vi "PicoHandsOnExample.vi"() -> ()   [LabVIEW 2020]
doc: "Example that shows how to communicate with the Hands On Raspberry Pico board used during the CTI LabVIEW Training"
uses:
  <instrlib>/HandsOnPi2040/Public/DigIns.ctl
  <instrlib>/HandsOnPi2040/Public/AnaIns.ctl
  <instrlib>/HandsOnPi2040/Public/DigOuts.ctl
  <instrlib>/HandsOnPi2040/cti-drivers-lv-visa-main/CTI-Visa/Identity.ctl
  <instrlib>/HandsOnPi2040/Public/AOs.ctl
  <instrlib>/HandsOnPi2040/Public/PWMSettings.ctl
  <instrlib>/HandsOnPi2040/HandsOnPi2040.lvlib
  <instrlib>/HandsOnPi2040/cti-drivers-lv-visa-main/CTI-Visa/CTI-Visa.lvlib
panel:
  in  "Frequency":sgl(slide) scale=10.0..500000.0
  in  "Duty":sgl(slide) scale=0.0..1.0
  out "Identity":T1
  out "LoopIndex":i32
  in  "Digital Output":T2=enum."DO1 (GPIO2)"
  in  "DOBEEP":bool
  in  "DO4":bool
  in  "DO3":bool
  in  "DO2":bool
  out "AnInValue":u16(graph)
  in  "Analog Inputs":T3=enum."AI1 (GPIO26)"
  out "DIStatus":bool
  in  "Digital Inputs":T4=enum."DI1 (GPIO7)"
  out "DOStatus":bool
  in  "DO1":bool
  in  "VISA resource name":refnum<visa-resource-name>="TCPIP0::192.168.10.207::6430::SOCKET"
  out "error out":errorcluster
  in  "stop":bool
  # "READ"
  # "WRITE"
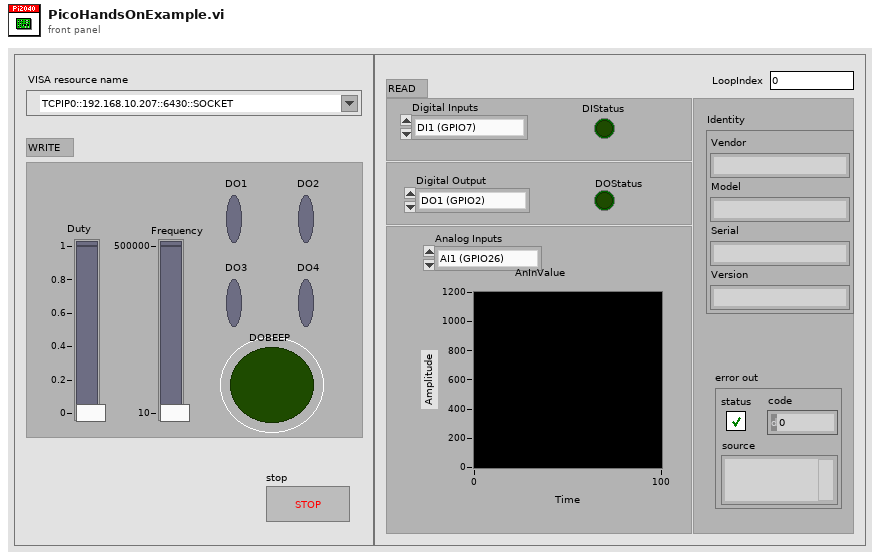
[diagram p1: front panel]
types:
  T1 = typedef "CTI-Visa.lvlib/Identity.ctl" = cluster{"Vendor":string, "Model":string, "Serial":string, "Version":string}
  T2 = typedef "HandsOnPi2040.lvlib/DigOuts.ctl" = enum16{"No DO - Error", "DO1 (GPIO2)", "DO2 (GPIO3)", "DO3 (GPIO4)", "DO4 (GPIO5)", "BEEP (GPIO6)"}
  T3 = typedef "HandsOnPi2040.lvlib/AnaIns.ctl" = enum16{"No AI - Error", "AI1 (GPIO26)", "AI2 (GPIO27)"}
  T4 = typedef "HandsOnPi2040.lvlib/DigIns.ctl" = enum16{"No DI - Error", "DI1 (GPIO7)", "DI2 (GPIO8)", "DI3 (GPIO9)", "DI4 (GPIO10)"}
  T5 = typedef "HandsOnPi2040.lvlib/PWMSettings.ctl" = cluster{"Duty":sgl, "Frequency":sgl}
  T6 = typedef "HandsOnPi2040.lvlib/AOs.ctl" = enum16{"No AO - Error", "AO1 (GPIO28)"}
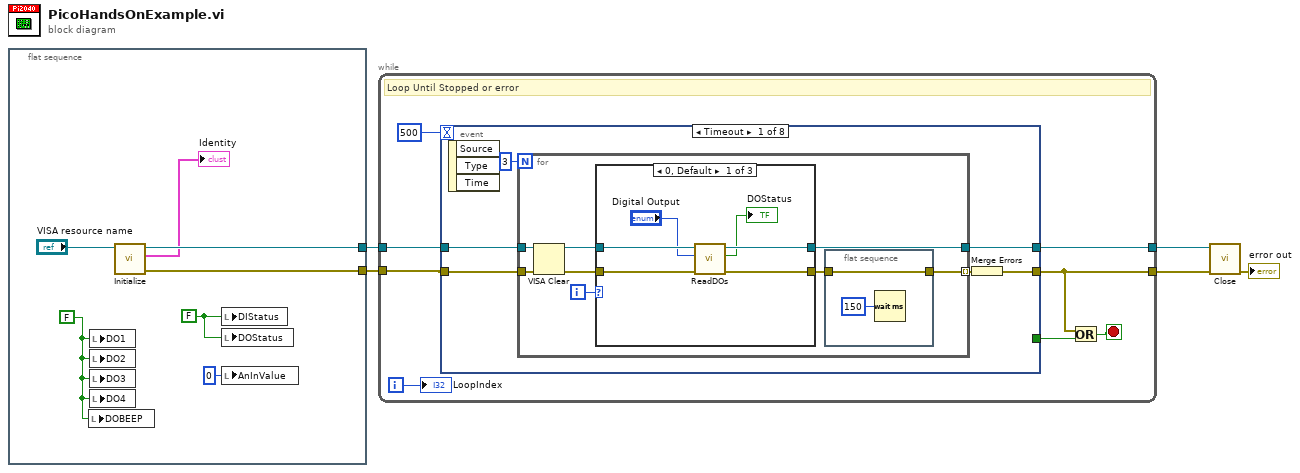
[diagram p0: block diagram]
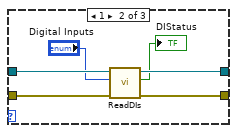
[diagram p2: hidden frame]
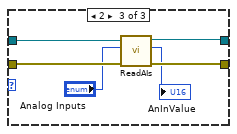
[diagram p3: hidden frame]
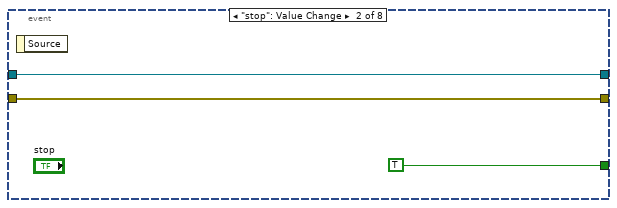
[diagram p4: hidden frame]
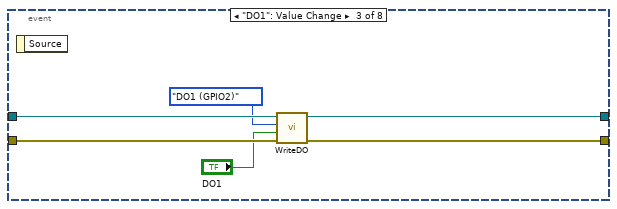
[diagram p5: hidden frame]
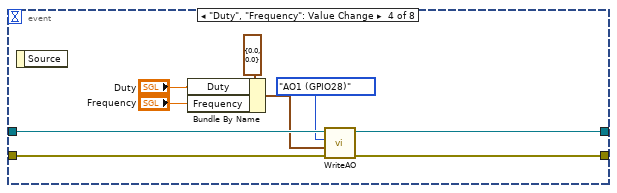
[diagram p6: hidden frame]
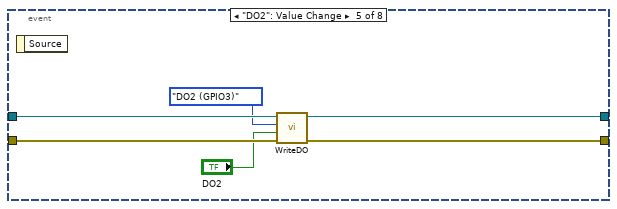
[diagram p7: hidden frame]
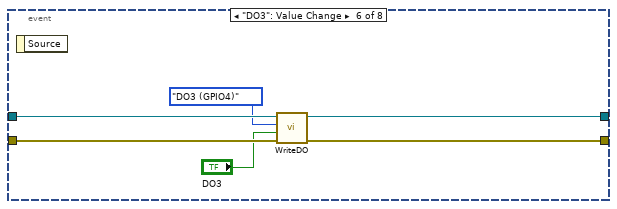
[diagram p8: hidden frame]
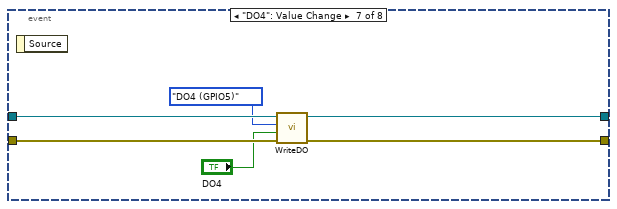
[diagram p9: hidden frame]
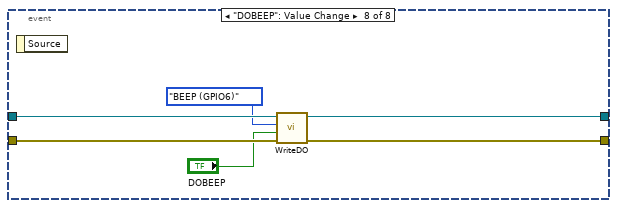
[diagram p10: hidden frame]
diagram:
  n1 = flat-sequence {
    tunnel: [w11] -> w2
    tunnel: [w10] -> w1
    frame #0 {
      w6 = FALSE ("WriteAnOut")
      w9 = FALSE ("WriteAnOut")
      n2 = local write "DOBEEP"(w9) -> ()
      n3 = local write "DO1"(w9) -> ()
      n4 = local write "DO2"(w9) -> ()
      n5 = local write "DO3"(w9) -> ()
      n6 = local write "DO4"(w9) -> ()
      n7 = call <instrlib>:"Initialize.vi"("VISA resource name"="VISA resource name") -> ("error out"=w10:errorcluster, "Identity"=→"Identity":T1, "VISA resource name out"=w11:refnum<visa-resource-name>)  [unwired: 8 in]
      n8 = local write "DIStatus"(w6) -> ()
      n9 = local write "DOStatus"(w6) -> ()
      n10 = local write "AnInValue"(u16 0 ("AnInValue")) -> ()
    }
  }
  n11 = while {
    tunnel: [w15] -> w5
    tunnel: w2 -> [w20]
    tunnel: [w19] -> w3
    tunnel: w1 -> [w17]
    i -> [w16]
    stop <- w13 stop-if-true
    # "Loop Until Stopped or error"
    n12 = event shown="[0] Timeout" {
      selector: _ -> [_ _ _ _ _ _ _ _]
      dyn-events: _ -> [_ _ _ _ _ _ _ _]
      timeout: 500 -> [_ _ _ _ _ _ _ _]
      tunnel: [_ TRUE _ _ _ _ _ _] -> w14
      tunnel: [w24 w54 w62 w68 w77 w83 w89 w95] -> w15
      tunnel: w17 -> [w26 w54 w61 w70 w76 w82 w88 w94]
      tunnel: w20 -> [w23 w55 w60 w71 w75 w81 w87 w93]
      tunnel: [w22 w55 w59 w69 w74 w80 w86 w92] -> w19
      event Timeout {
        n13 = event-data() -> ()  [unwired: 1 in, 3 out]
        n14 = for {
          N: 3 -> [_]
          tunnel: w26 -> [w32]
          tunnel: [w28] -> w25 mode=indexing
          tunnel: w23 -> [w31]
          tunnel: [w30] -> w22
          i -> [w33]
          n15 = VISA Clear(VISA resource name=w31) -> (VISA resource name out=w27:refnum<visa-resource-name>)  [unwired: 1 in, 1 out]
          n16 = case shown="0, Default" w33 {
            tunnel: w32 -> [w41 w46 w52]
            tunnel: [w40 w44 w50] -> w29
            tunnel: w27 -> [w39 w47 w53]
            tunnel: [w38 w45 w51] -> w30
            frame 0, Default {
              n17 = call <instrlib>:"ReadDOs.vi"("error in (no error)"=w41, "Output"="Digital Output", "VISA resource name"=w39) -> ("error out"=w40:errorcluster, "DOStatus"=→"DOStatus":bool, "VISA resource name out"=w38:refnum<visa-resource-name>)  [unwired: 6 in]
            }
            frame 1 {
              n18 = call <instrlib>:"ReadDIs.vi"("error in (no error)"=w46, "Digital Inputs"="Digital Inputs", "VISA resource name"=w47) -> ("error out"=w44:errorcluster, "DIStatus"=→"DIStatus":bool, "VISA resource name out"=w45:refnum<visa-resource-name>)  [unwired: 6 in]
            }
            frame 2 {
              n19 = call <instrlib>:"ReadAIs.vi"("error in (no error)"=w52, "Analog Inputs"="Analog Inputs", "VISA resource name"=w53) -> ("error out"=w50:errorcluster, "Value"=→"AnInValue":u16, "VISA resource name out"=w51:refnum<visa-resource-name>)  [unwired: 6 in]
            }
          }
          n20 = flat-sequence {
            tunnel: w29 -> [w35]
            tunnel: [w35] -> w28
            frame #0 {
              n21 = Wait (ms)(milliseconds to wait=u32 150) -> ()  [unwired: 1 out]
            }
          }
        }
        n22 = Merge Errors(w25) -> (w24:errorcluster)
      }
      event "stop": Value Change {
        n23 = event-data() -> ()  [unwired: 1 in, 1 out]
      }
      event "DO1": Value Change {
        n24 = event-data() -> ()  [unwired: 1 in, 1 out]
        n25 = call <instrlib>:"WriteDO.vi"("error in (no error)"=w61, "DO Value (True)"="DO1", "Output"=DigOuts."DO1 (GPIO2)" ("Write Digital Output"), "VISA resource name"=w60) -> ("error out"=w62:errorcluster, "VISA resource name out"=w59:refnum<visa-resource-name>)  [unwired: 6 in]
      }
      event "Duty", "Frequency": Value Change {
        n26 = event-data() -> ()  [unwired: 1 in, 1 out]
        n27 = Bundle By Name(cluster=T5 {"Duty"=0.0, "Frequency"=0.0} ("PWM Settings"), "Duty"="Duty", "Frequency"="Frequency") -> (w65:T5)
        n28 = call <instrlib>:"WriteAO.vi"("error in (no error)"=w70, "PWM Settings"=w65, "Analog Output"=AOs."AO1 (GPIO28)", "VISA resource name"=w71) -> ("error out"=w68:errorcluster, "VISA resource name out"=w69:refnum<visa-resource-name>)  [unwired: 6 in]
      }
      event "DO2": Value Change {
        n29 = event-data() -> ()  [unwired: 1 in, 1 out]
        n30 = call <instrlib>:"WriteDO.vi"("error in (no error)"=w76, "DO Value (True)"="DO2", "Output"=DigOuts."DO2 (GPIO3)" ("Write Digital Output"), "VISA resource name"=w75) -> ("error out"=w77:errorcluster, "VISA resource name out"=w74:refnum<visa-resource-name>)  [unwired: 6 in]
      }
      event "DO3": Value Change {
        n31 = event-data() -> ()  [unwired: 1 in, 1 out]
        n32 = call <instrlib>:"WriteDO.vi"("error in (no error)"=w82, "DO Value (True)"="DO3", "Output"=DigOuts."DO3 (GPIO4)" ("Write Digital Output"), "VISA resource name"=w81) -> ("error out"=w83:errorcluster, "VISA resource name out"=w80:refnum<visa-resource-name>)  [unwired: 6 in]
      }
      event "DO4": Value Change {
        n33 = event-data() -> ()  [unwired: 1 in, 1 out]
        n34 = call <instrlib>:"WriteDO.vi"("error in (no error)"=w88, "DO Value (True)"="DO4", "Output"=DigOuts."DO4 (GPIO5)" ("Write Digital Output"), "VISA resource name"=w87) -> ("error out"=w89:errorcluster, "VISA resource name out"=w86:refnum<visa-resource-name>)  [unwired: 6 in]
      }
      event "DOBEEP": Value Change {
        n35 = event-data() -> ()  [unwired: 1 in, 1 out]
        n36 = call <instrlib>:"WriteDO.vi"("error in (no error)"=w94, "DO Value (True)"="DOBEEP", "Output"=DigOuts."BEEP (GPIO6)" ("Write Digital Output"), "VISA resource name"=w93) -> ("error out"=w95:errorcluster, "VISA resource name out"=w92:refnum<visa-resource-name>)  [unwired: 6 in]
      }
    }
    n37 = Or(x=w15, y=w14) -> (x .or. y?=w13:bool)
    "LoopIndex" <- w16
  }
  n38 = call <instrlib>:"Close.vi"("error in (no error)"=w5, "VISA resource name"=w3) -> ("error out"=→"error out":errorcluster)  [unwired: 9 in]
